vi "Register Stop Battle Event.vi"(8 "error in (no error)":errorcluster, 10 "Stop Battle":refnum<user-event>, 11 "Dashboard Panel in":refnum<class "Dashboard Panel.lvclass">) -> (0 "error out":errorcluster, 3 "Dashboard Panel out":refnum<class "Dashboard Panel.lvclass">)   [LabVIEW 2020, in "SB App.lvlib" / "Dashboard Panel.lvclass"]
uses:
  Dashboard Panel.lvclass
  Dashboard Panel.lvclass/Dashboard Panel.ctl
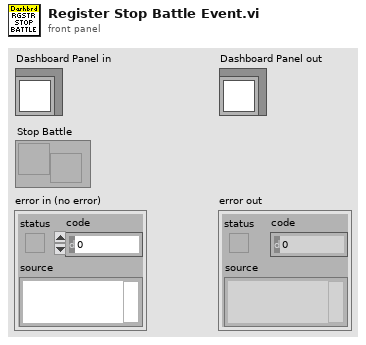
[diagram p1: front panel]
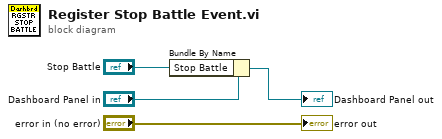
[diagram p0: block diagram]
diagram:
  n1 = Bundle By Name(cluster="Dashboard Panel in", "Stop Battle"="Stop Battle") -> (→"Dashboard Panel out":refnum<class "Dashboard Panel.lvclass">)
  "error out" <- "error in (no error)"
